vi "(SubVI) Optimizing text height.vi"(1 "comp space":u32, 2 "content comp arr":refnum<vi>[](array[refnum])) -> ()   [LabVIEW 2022 SP3]
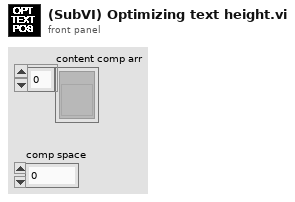
[diagram p1: front panel]
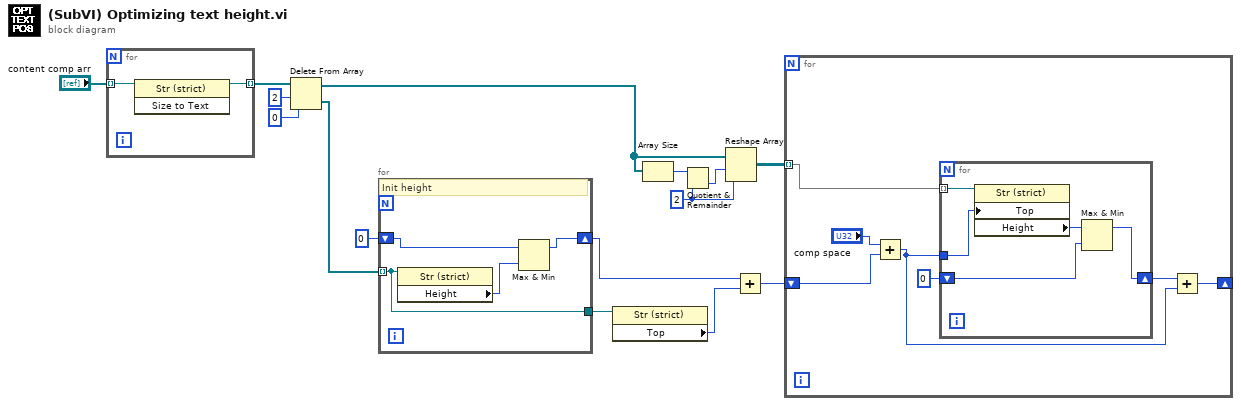
[diagram p0: block diagram]
diagram:
  w15 = 2 ("y")
  n1 = for {
    tunnel: "content comp arr" -> [w17] mode=indexing
    tunnel: [w16] -> w6 mode=indexing
    n2 = invoke class="Str (strict)" method="Size to Text"(reference=w17) -> (reference out=w16:refnum<vi>)  [unwired: 2 in, 2 out]
  }
  n3 = Delete From Array(array=w6, length=2, index=0) -> (deleted portion=w8:refnum<vi>[], array with subset deleted=w9:refnum<vi>[])
  n4 = for {
    shift-right: [w19] -> w3
    shift-left: 0 ("index (row)") -> [w21]
    tunnel: w8 -> [w18] mode=indexing
    tunnel: [w18] -> w5
    # "Init height"
    n5 = property class="Str (strict)"(reference=w18) -> ("Height"=w20:u32)  [unwired: 1 in, 2 out]
    n6 = Max & Min(x=w21, y=w20) -> (max(x,y)=w19:u32)  [unwired: 1 out]
  }
  n7 = property class="Str (strict)"(reference=w5) -> ("Top"=w4:i32)  [unwired: 1 in, 2 out]
  n8 = Array Size(array=w9) -> (size(s)=w13:i32)
  n9 = Quotient & Remainder(x=w13, y=w15) -> (floor(x/y)=w14:i32)  [unwired: 1 out]
  n10 = Reshape Array(w9, w14, w15) -> (w2:refnum<vi>[][])
  n11 = Add(x=w3, y=w4) -> (x+y=w1:u32)
  n12 = for {
    tunnel: w2 -> [w26] mode=indexing
    shift-right: [w22] -> _
    shift-left: w1 -> [w27]
    n13 = Add(x="comp space", y=w27) -> (x+y=w23:u32)
    n14 = for {
      tunnel: w26 -> [w33] mode=indexing
      tunnel: w23 -> [w32]
      shift-right: [w29] -> w24
      shift-left: 0 ("index (row)") -> [w30]
      n15 = property class="Str (strict)"(reference=w33, "Top"=w32) -> ("Height"=w31:u32)  [unwired: 1 in, 2 out]
      n16 = Max & Min(x=w31, y=w30) -> (max(x,y)=w29:u32)  [unwired: 1 out]
    }
    n17 = Add(x=w24, y=w23) -> (x+y=w22:u32)
  }
